vi "Generate Observer Message Set.vi"(9 "Mediator Enqueuer":refnum<class "Message Enqueuer.lvclass">, 11 "Mediator Type":refnum<class "IMediator.lvclass">) -> (2 "Unsubscribe Msg":refnum<class "Unsubscribe Msg.lvclass">, 3 "Subscribe Msg":refnum<class "Subscribe Msg.lvclass">)   [LabVIEW 2019, in "IMediator.lvlib" / "IMediator.lvclass"]
uses:
  <vilib>/gpm_packages/@cs/mva-core/Source/IMediator/IMediator/IMediator.lvclass
  <vilib>/gpm_packages/@cs/mva-core/Source/IMediator/IMediator Messages/Subscribe Msg/Subscribe Msg.lvclass
  C:/Program Files/National Instruments/LabVIEW 2019/vi.lib/gpm_packages/@cs/actor-framework-messages/Source/RoundTripMessage/RoundTripMessage.lvclass
  <vilib>/gpm_packages/@cs/mva-core/Source/IMediator/IMediator Messages/Unsubscribe Msg/Unsubscribe Msg.lvclass
  <vilib>/ActorFramework/Message Enqueuer/Message Enqueuer.lvclass
  <vilib>/gpm_packages/@cs/actor-framework-messages/Source/RoundTripMessage/RoundTripMessage.lvclass/RoundTripMessage.ctl
  <vilib>/gpm_packages/@cs/actor-framework-messages/Source/RoundTripMessage/Write Return Address.vi
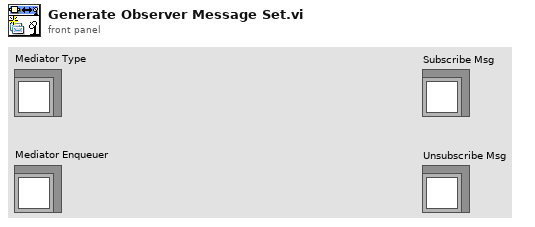
[diagram p1: front panel]
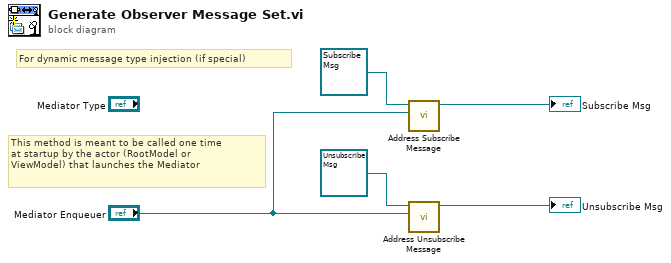
[diagram p0: block diagram]
diagram:
  # "This method is meant to be called one time\nat startup by the actor (RootModel or\nViewModel) that launches the Mediator"
  # "For dynamic message type injection (if special)"
  n1 = call <vilib>:"Address Subscribe Message.vi"("Mediator Enqueuer"="Mediator Enqueuer", "Subscribe Msg In"=refnum<class "Subscribe Msg.lvclass"> refnum) -> ("Subscribe Msg Out"=→"Subscribe Msg":refnum<class "Subscribe Msg.lvclass">)  [unwired: 9 in]
  n2 = call <vilib>:"Address Unsubscribe Message.vi"("Mediator Enqueuer"="Mediator Enqueuer", "Unsubscribe Msg In"=refnum<class "Unsubscribe Msg.lvclass"> refnum) -> ("Unsubscribe Msg Out"=→"Unsubscribe Msg":refnum<class "Unsubscribe Msg.lvclass">)  [unwired: 9 in]
